vi "Pre-Reanimate Hook.vi"(8 "Error In":errorcluster) -> (0 "Error Out":errorcluster)   [LabVIEW 2018, in "Tests.lvlib" / "Toolkit.lvlib" / "Integration.lvlib"]
uses:
  Integration.lvlib
  Hooks/Pre-Reanimate.vi
  Support/Reanimate Target.vi
  <vilib>/addons/_JKI Toolkits/Caraya/classes/Test/Test.lvclass
  Tests.lvlib
  <vilib>/addons/_JKI Toolkits/Caraya/classes/Assert/Assert.lvclass
  src/Toolkit/Toolkit.lvlib
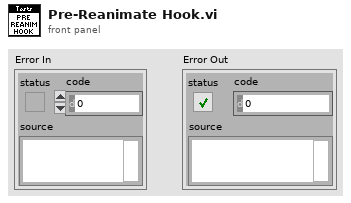
[diagram p1: front panel]
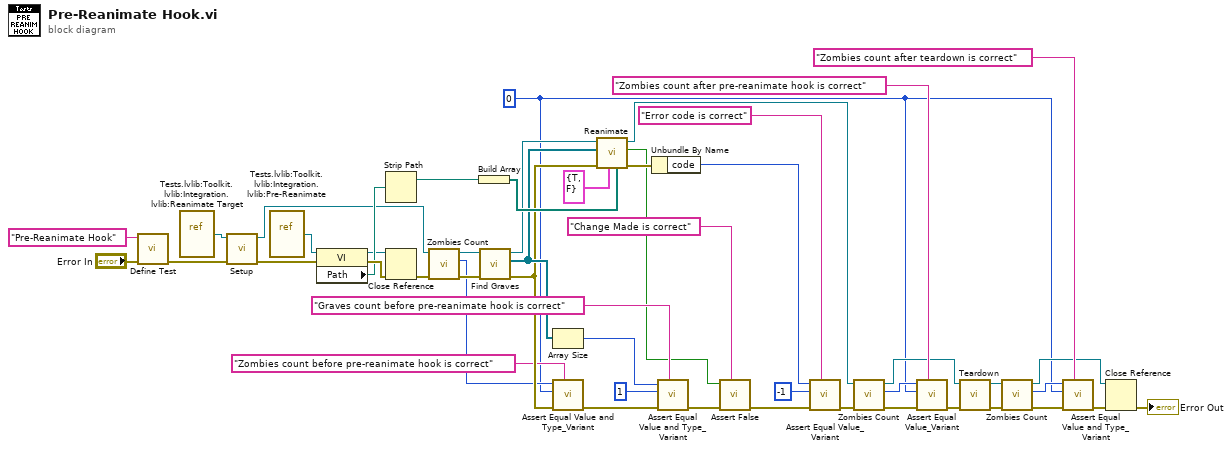
[diagram p0: block diagram]
diagram:
  w1 = 0 ("size(s)")
  n1 = call <vilib>:"Define Test.vi"("error in (no error)"="Error In", "Label (VI Title)"="Pre-Reanimate Hook") -> ("error out"=w44:errorcluster)  [unwired: 9 in]
  n2 = vi-ref "Tests.lvlib:Toolkit.lvlib:Integration.lvlib:Reanimate Target.vi"() -> (w10:refnum<vi>)
  n3 = call "Setup.vi"("Error In"=w44, "VI In"=w10) -> ("Error Out"=w34:errorcluster, "VI Out"=w26:refnum<vi>)  [unwired: 8 in]
  n4 = vi-ref "Tests.lvlib:Toolkit.lvlib:Integration.lvlib:Pre-Reanimate.vi"() -> (w11:refnum<vi>)
  n5 = property class="VI"(reference=w11, error in=w34) -> (reference out=w30:refnum<vi>, error out=w33:errorcluster, "Path"=w32:path)
  n6 = Strip Path(path=w32) -> (stripped path=w31:path)  [unwired: 1 out]
  n7 = Close Reference(reference=w30, error in (no error)=w33) -> (error out=w7:errorcluster)
  n8 = call "Zombies Count.vi"("Error In"=w7, "Test Target In"=w26) -> ("Error Out"=w6:errorcluster, "Zombies Count"=w2:i32, "Test Target Out"=w8:refnum<vi>)  [unwired: 7 in]
  n9 = Build Array(w31) -> (w27:path[])
  n10 = call "Find Graves.vi"("Error In"=w6, "VI In"=w8) -> ("Error Out"=w5:errorcluster, "Graves"=w24:refnum<vi>[], "VI Out"=w25:refnum<vi>)  [unwired: 7 in]
  n11 = Array Size(array=w24) -> (size(s)=w23:i32)
  n12 = call <vilib>:"Assert Equal Value and Type_Variant.vi"("Label"="Zombies count before pre-reanimate hook is correct", "error in (no error)"=w5, "Y"=w1, "X"=w2) -> ("error out"=w4:errorcluster)  [unwired: 7 in]
  n13 = call "Reanimate.vi"("Hook Search Path"=w27, "Execute Hooks?"=cluster{"Pre":bool, "Post":bool} {"Pre"=TRUE, "Post"=FALSE}, "Error In"=w5, "Graves"=w24, "VI In"=w25) -> ("Error Out"=w22:errorcluster, "Change Made?"=w13:bool, "VI Out"=w17:refnum<vi>)  [unwired: 4 in]
  n14 = Unbundle By Name(w22) -> ("code"=w29:i32)
  n15 = call <vilib>:"Assert Equal Value and Type_Variant.vi"("Label"="Graves count before pre-reanimate hook is correct", "error in (no error)"=w4, "Y"=1 ("size(s)"), "X"=w23) -> ("error out"=w43:errorcluster)  [unwired: 7 in]
  n16 = call <vilib>:"Assert False.vi"("Label"="Change Made is correct", "error in (no error)"=w43, "False?"=w13) -> ("error out"=w14:errorcluster)  [unwired: 8 in]
  n17 = call <vilib>:"Assert Equal Value_Variant.vi"("Label"="Error code is correct", "error in (no error)"=w14, "Y"=-1 ("code"), "X"=w29) -> ("error out"=w21:errorcluster)  [unwired: 7 in]
  n18 = call "Zombies Count.vi"("Error In"=w21, "Test Target In"=w17) -> ("Error Out"=w20:errorcluster, "Zombies Count"=w19:i32, "Test Target Out"=w18:refnum<vi>)  [unwired: 7 in]
  n19 = call <vilib>:"Assert Equal Value_Variant.vi"("Label"="Zombies count after pre-reanimate hook is correct", "error in (no error)"=w20, "Y"=w1, "X"=w19) -> ("error out"=w16:errorcluster)  [unwired: 7 in]
  n20 = call "Teardown.vi"("Error In"=w16, "VI In"=w18) -> ("Error Out"=w37:errorcluster, "VI Out"=w39:refnum<vi>)  [unwired: 8 in]
  n21 = call "Zombies Count.vi"("Error In"=w37, "Test Target In"=w39) -> ("Error Out"=w36:errorcluster, "Zombies Count"=w35:i32, "Test Target Out"=w38:refnum<vi>)  [unwired: 7 in]
  n22 = call <vilib>:"Assert Equal Value and Type_Variant.vi"("Label"="Zombies count after teardown is correct", "error in (no error)"=w36, "Y"=w1, "X"=w35) -> ("error out"=w41:errorcluster)  [unwired: 7 in]
  n23 = Close Reference(reference=w38, error in (no error)=w41) -> (error out=→"Error Out":errorcluster)
